vi "LaserCal-Initialize (I-O).vi"(0 "Stimulus":T4, 5 "Taverage (ms)":dbl, 9 "Response params":T2, 11 "error in (no error)":errorcluster) -> (4 "Runtime State":T3={"AO Channels"=[], "Fs (Hz)"=100000.0, "Npts"=1, "conversion"=0.0}, 8 "SeqVars":dbl[](array[numeric]), 14 "I-O Data":T1, 15 "error out":errorcluster)   [LabVIEW 2015]
uses:
  Typedefs/LaserCal-IO Stimulus Params.ctl
  Typedefs/LaserCal-Meter Runtime State.ctl
  Typedefs/LaserCal-IO Response Params.ctl
  Typedefs/LaserCal-Data (I-O).ctl
panel:
  in  "T (s)":dbl=1.0
  in  "Fs (Hz)":dbl=100000.0
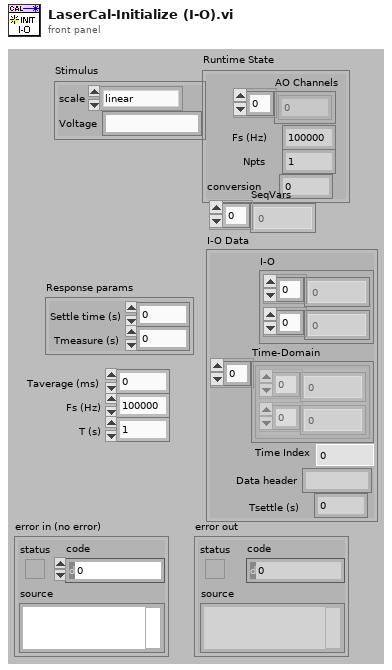
[diagram p1: front panel]
types:
  T1 = typedef "LaserCal-Data (I-O).ctl" = cluster{"I-O":cluster{dbl[], dbl[]}, "Time-Domain":cluster{dbl[], dbl[]}[], "Time Index":i32, "Data header":string, "Tsettle (s)":dbl}
  T2 = typedef "LaserCal-IO Response Params.ctl" = cluster{"Settle time (s)":dbl, "Tmeasure (s)":dbl}
  T3 = typedef "LaserCal-Meter Runtime State.ctl" = cluster{"AO Channels":i32[], "Fs (Hz)":dbl, "Npts":i32, "conversion":dbl}
  T4 = typedef "LaserCal-IO Stimulus Params.ctl" = cluster{"scale":enum16{"linear", "dB"}, "Voltage":string}
  T5 = cluster{cluster{"Array":dbl[], dbl[]}, cluster{dbl[], dbl[]}[], i32, "header":string, dbl}
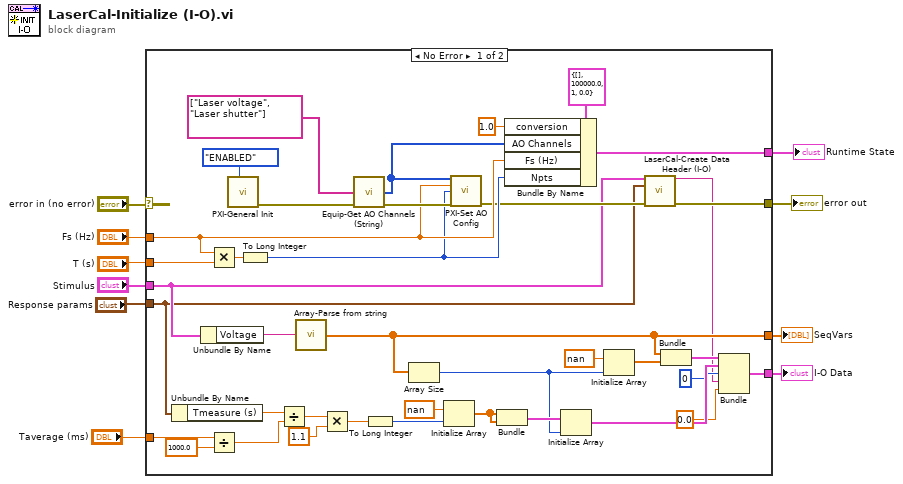
[diagram p0: block diagram]
diagram:
  n1 = case shown="No Error" "error in (no error)" {
    selector: "error in (no error)" -> [_ w49]
    tunnel: [w15 w49] -> w9
    tunnel: "Fs (Hz)" -> [w40 _]
    tunnel: "T (s)" -> [w44 _]
    tunnel: "Stimulus" -> [w14 _]
    tunnel: [w38 _] -> w5
    tunnel: [w23 _] -> w4
    tunnel: "Response params" -> [w13 _]
    tunnel: "Taverage (ms)" -> [w36 _]
    tunnel: [w18 _] -> w1
    frame No Error {
      n2 = Unbundle By Name(w13) -> ("Tmeasure (s)"=w34:dbl)
      n3 = Unbundle By Name(w14) -> ("Voltage"=w37:string)
      n4 = Multiply(x=w40, y=w44) -> (x*y=w43:dbl)
      n5 = Divide(x=w36, y=1000.0) -> (x/y=w33:dbl)
      n6 = call "PXI-General Init.vi"("Double Buffer Mode"=enum32{"OFF", "ENABLED", "FORCED"}."ENABLED") -> ("error out"=w47:errorcluster)  [unwired: 10 in]
      n7 = To Long Integer(number=w43) -> (32bit integer=w39:i32)
      n8 = Divide(x=w34, y=w33) -> (x/y=w32:dbl)
      n9 = call "Array-Parse from string.vi"("String"=w37) -> ("Array"=w23:dbl[])  [unwired: 13 in, 1 out]
      n10 = Multiply(x=w32, y=1.1) -> (x*y=w30:dbl)
      n11 = call "Equip-Get AO Channels (String).vi"("Channel Names"=string[] ["Laser voltage", "Laser shutter"], "error in (no error)"=w47) -> ("AO Channels"=w41:i32[], "error out"=w46:errorcluster)  [unwired: 12 in]
      n12 = To Long Integer(number=w30) -> (32bit integer=w29:i32)
      n13 = Array Size(array=w23) -> (size(s)=w24:i32)
      n14 = Initialize Array(nan ("element"), w29) -> (w27:dbl[])
      n15 = call "PXI-Set AO Config.vi"("AO Channels"=w41, "Sampling Rate (Hz)"=w40, "Buffer Size"=w39, "error in (no error)"=w46) -> ("error out"=w16:errorcluster)  [unwired: 11 in]
      n16 = Bundle(w27, w27) -> (w26:cluster{dbl[], dbl[]})  [unwired: 1 in]
      n17 = Bundle By Name(cluster=T3 {"AO Channels"=[], "Fs (Hz)"=100000.0, "Npts"=1, "conversion"=0.0} ("Runtime State"), "conversion"=1.0, "AO Channels"=w41, "Fs (Hz)"=w40, "Npts"=w39) -> (w38:T3)
      n18 = Initialize Array(w26, w24) -> (w20:cluster{dbl[], dbl[]}[])
      n19 = Initialize Array(nan ("element"), w24) -> (w22:dbl[])
      n20 = call "LaserCal-Create Data Header (I-O).vi"("Stimulus"=w14, "Response params"=w13, "error in (no error)"=w16) -> ("header"=w12:string, "error out"=w15:errorcluster)  [unwired: 11 in]
      n21 = Bundle("Array"=w23, w22) -> (w21:cluster{"Array":dbl[], dbl[]})  [unwired: 1 in]
      n22 = Bundle(w21, w20, 0, "header"=w12, 0.0) -> (w18:T5)  [unwired: 1 in]
    }
    frame Error {
    }
  }
  "error out" <- w9
  "Runtime State" <- w5
  "SeqVars" <- w4
  "I-O Data" <- w1
